vi "Configure Square Duty Cycle.vi"(8 "error in (no error)":errorcluster, 10 "Duty Cycle (50 %)":i32=50 min=0 max=100, 11 "VISA resource name":refnum<visa-resource-name>) -> (0 "error out":errorcluster, 3 "VISA resource name out":refnum<visa-resource-name>)   [LabVIEW 2017, in "Keithley 3390.lvlib"]
doc: "Sets the duty cycle of the square waveform."
uses:
  Keithley 3390.lvlib
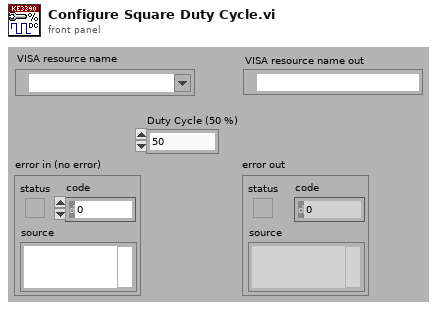
[diagram p1: front panel]
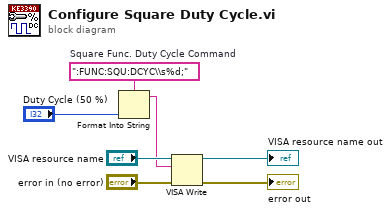
[diagram p0: block diagram]
diagram:
  w3 = ":FUNC:SQU:DCYC\\s%d;"  # Square Func. Duty Cycle Command
  n1 = Format Into String(format string=w3, "Duty Cycle (50 %)") -> (resulting string=w5:string)  [unwired: 2 in, 1 out]
  n2 = VISA Write(VISA resource name="VISA resource name", write buffer=w5, error in (no error)="error in (no error)") -> (VISA resource name out=→"VISA resource name out":refnum<visa-resource-name>, error out=→"error out":errorcluster)  [unwired: 1 out]
